vi "Beeper.vi"(3 "error in (no error)":errorcluster, 4 "Number of Tones (Def=4)":i32=4) -> (0 "error (thru)":errorcluster)   [LabVIEW 2020]
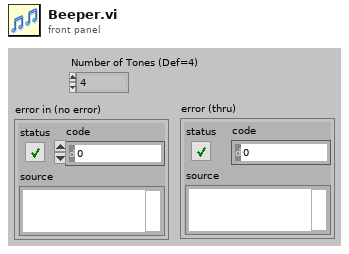
[diagram p1: front panel]
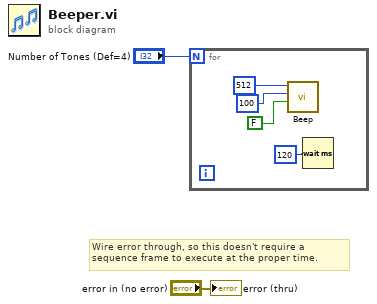
[diagram p0: block diagram]
diagram:
  # "Wire error through, so this doesn't require a sequence frame to execute at the proper time."
  n1 = for {
    N: "Number of Tones (Def=4)" -> [_]
    n2 = call <vilib>:"Beep.vi"("use system alert? (T)"=FALSE, "duration (msec)"=100, "frequency (Hz)"=512) -> ()  [unwired: 9 in]
    n3 = Wait (ms)(milliseconds to wait=120) -> ()  [unwired: 1 out]
  }
  "error (thru)" <- "error in (no error)"
